vi "Labels In Structures.vi"   [LabVIEW 2019]
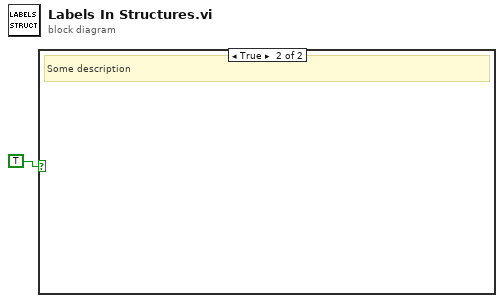
[diagram p0: block diagram]
diagram:
  n1 = case shown="True" TRUE {
    frame False {
    }
    frame True {
      # "Some description"
    }
  }
